vi "Get JSON Data.vi"(6 "Force Hide":bool, 7 "Evaluate Pane Move":bool, 8 "error in (no error)":errorcluster, 9 "Force Get All Data":bool, 10 "VI Reference":refnum<vi>, 11 "Numeric In":refnum<class "Numeric.lvclass">) -> (0 "error out":errorcluster, 2 "JSON string":string, 3 "Numeric Out":refnum<class "Numeric.lvclass">)   [LabVIEW 2017, in "Front Panel Publisher.lvlib" / "Numeric.lvclass"]
uses:
  Numeric.lvclass
  Control_class/Control.lvclass
  Object_class/Object.lvclass
  Web Front Panel_class/Controls/Enum - Control Display Mode.ctl
  Web Front Panel_class/Web Front Panel.lvclass
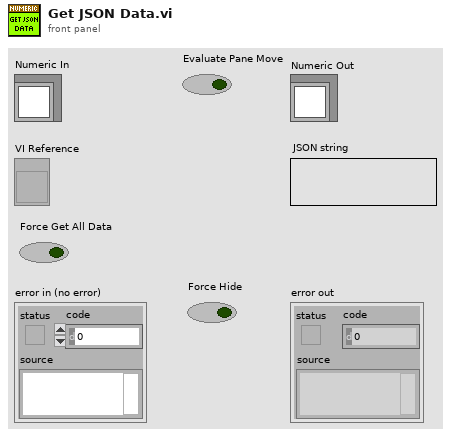
[diagram p1: front panel]
types:
  T1 = typedef "Front Panel Publisher.lvlib/Web Front Panel.lvclass/Enum - Control Display Mode.ctl" = enum16{"Value Only", "Value and Visibility", "Boolean Value Only", "Boolean Value and Visibility", "Control is Image", "Image and Visibility"}
  T2 = typedef "Front Panel Publisher.lvlib/Object.lvclass/Attributes.ctl" = cluster{"UID":i32, "Type":string, "Starting Location":T3, "Reference":refnum<vi>, "Cluster Component":bool, "Starting Rect Position":cluster{"Left":i16, "Top":i16}, "Owning Pane":refnum<vi>, "Master Total Rect Delta":T4}
  T3 = typedef "Front Panel Publisher.lvlib/Object.lvclass/Coordinates.ctl" = cluster{"Left":i32, "Top":i32, "Height":u32, "Width":u32}
  T4 = typedef "LVRectTypeDef.ctl" = cluster{"Left":i16, "Top":i16, "Right":i16, "Bottom":i16}
  T5 = typedef "Front Panel Publisher.lvlib/Control.lvclass/Attributes.ctl" = cluster{"Description":string, "Indicator":bool, "Default Value":variant, "Control Index":i32, "Label":refnum<class "Text.lvclass">, "Caption":refnum<class "Text.lvclass">, "Image b64":string, "No Control Index":bool, "Display Mode":T1}
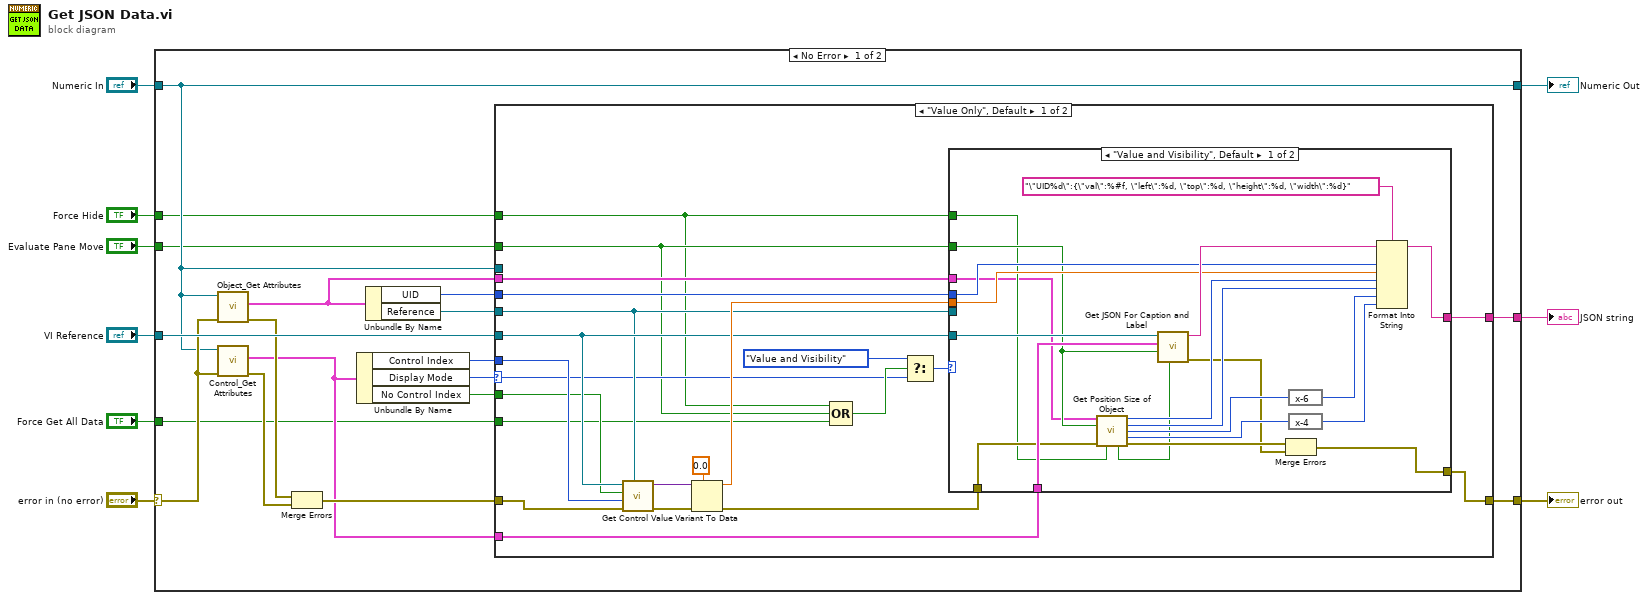
[diagram p0: block diagram]
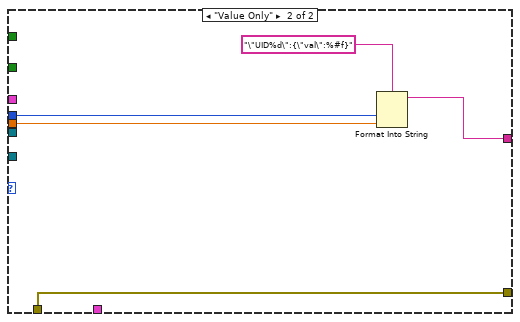
[diagram p2: hidden frame]
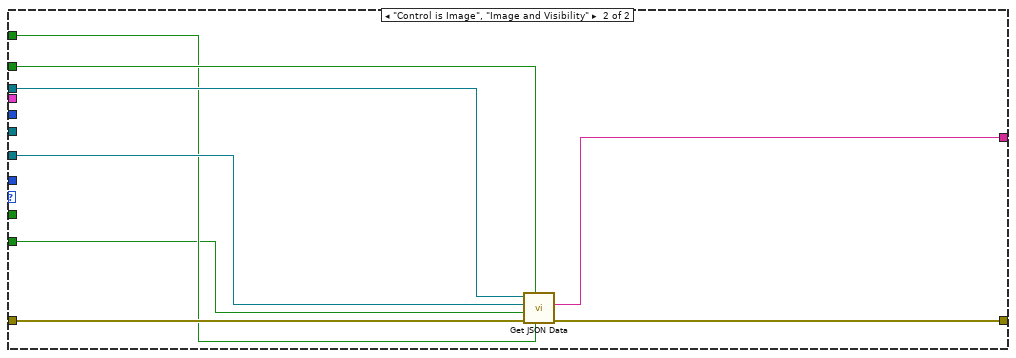
[diagram p3: hidden frame]
diagram:
  n1 = case shown="No Error" "error in (no error)" {
    selector: "error in (no error)" -> [w22 w85]
    tunnel: [w19 w85] -> w8
    tunnel: [w16 w84] -> w6
    tunnel: "Numeric In" -> [w16 w84]
    tunnel: "VI Reference" -> [w25 _]
    tunnel: [w24 _] -> w4
    tunnel: "Force Get All Data" -> [w14 _]
    tunnel: "Evaluate Pane Move" -> [w13 _]
    tunnel: "Force Hide" -> [w11 _]
    frame No Error {
      n2 = call "Object_Get Attributes.vi"("error in (no error)"=w22, "Object In"=w16) -> ("error out"=w20:errorcluster, "Object Attributes"=w10:T2)  [unwired: 7 in, 1 out]
      n3 = call "Control_Get Attributes.vi"("error in (no error)"=w22, "Control In"=w16) -> ("error out"=w27:errorcluster, "Control Attributes"=w17:T5)  [unwired: 7 in, 1 out]
      n4 = Merge Errors(w20, w27) -> (w21:errorcluster)
      n5 = Unbundle By Name(w17) -> ("Control Index"=w26:i32, "Display Mode"=w18:T1, "No Control Index"=w12:bool)
      n6 = Unbundle By Name(w10) -> ("UID"=w23:i32, "Reference"=w15:refnum<vi>)
      n7 = case shown="\"Value Only\", Default" w18 {
        selector: w18 -> [w32 _]
        tunnel: w26 -> [w40 _]
        tunnel: w25 -> [w42 w79]
        tunnel: [w47 w82] -> w24
        tunnel: w23 -> [w46 _]
        tunnel: w21 -> [w39 w80]
        tunnel: [w43 w81] -> w19
        tunnel: w17 -> [w45 _]
        tunnel: w16 -> [_ w83]
        tunnel: w15 -> [w41 _]
        tunnel: w14 -> [w30 w76]
        tunnel: w13 -> [w29 w78]
        tunnel: w12 -> [w36 _]
        tunnel: w11 -> [w28 w77]
        tunnel: w10 -> [w35 _]
        frame "Value Only", Default {
          n8 = call "Get Control Value.vi"("Control Reference"=w41, "error in (no error)"=w39, "Control Index"=w40, "No Control Index"=w36, "VI Reference"=w42) -> ("error out"=w38:errorcluster, "Variant"=w37:variant)  [unwired: 5 in]
          n9 = Variant To Data(error in=w38, type=0.0, Variant=w37) -> (data=w48:dbl, error out=w44:errorcluster)
          n10 = Compound Arithmetic op=OR(w28, w29, w30) -> (w33:bool)
          n11 = Select(t=Enum_-_Control_Display_Mode."Value and Visibility", s=w33, f=w32) -> (s? t:f=w31:T1)
          n12 = case shown="\"Value and Visibility\", Default" w31 {
            tunnel: w48 -> [w61 w74]
            tunnel: [w60 w73] -> w47
            tunnel: w46 -> [w62 w72]
            tunnel: w45 -> [w59 _]
            tunnel: w41 -> [_ _]
            tunnel: w42 -> [w58 _]
            tunnel: w44 -> [w57 w71]
            tunnel: [w52 w71] -> w43
            tunnel: w29 -> [w55 _]
            tunnel: w28 -> [w54 _]
            tunnel: w35 -> [w50 _]
            frame "Value and Visibility", Default {
              n13 = call "Get Position Size of Object.vi"("Object Attributes"=w50, "Evaluate Pane Move"=w55, "error in (no error)"=w57, "Force Hide"=w54) -> ("Left"=w69:i32, "Top"=w68:i32, "Height"=w67:u32, "Width"=w66:u32, "Hidden"=w53:bool, "error out"=w56:errorcluster)  [unwired: 6 in]
              n14 = call "Get JSON For Caption and Label.vi"("Force Hide"=w53, "Evaluate Pane Move"=w55, "Data"=w59, "VI in"=w58) -> ("error out"=w51:errorcluster, "JSON"=w63:string)  [unwired: 6 in]
              n15 = Merge Errors(w56, w51) -> (w52:errorcluster)
              n16 = expression code="x-6"(w67) -> (w64:u32)
              n17 = expression code="x-4"(w66) -> (w65:u32)
              n18 = Format Into String(format string="\"UID%d\":{\"val\":%#f, \"left\":%d, \"top\":%d, \"height\":%d, \"width\":%d}", initial string=w63, w62, w61, w69, w68, w64, w65) -> (resulting string=w60:string)  [unwired: 1 in, 1 out]
            }
            frame "Value Only" {
              n19 = Format Into String(format string="\"UID%d\":{\"val\":%#f}", w72, w74) -> (resulting string=w73:string)  [unwired: 2 in, 1 out]
            }
          }
        }
        frame "Control is Image", "Image and Visibility" {
          n20 = call-parent "Get JSON Data.vi"("Force Hide"=w77, "Evaluate Pane Move"=w78, "error in (no error)"=w80, "Force Get All Data"=w76, "VI Reference"=w79, "Control In"=w83) -> ("error out"=w81:errorcluster, "JSON string"=w82:string)  [unwired: 3 in, 1 out]
        }
      }
    }
    frame Error {
    }
  }
  "error out" <- w8
  "Numeric Out" <- w6
  "JSON string" <- w4
